vi "CIMAQ_distance_map.vi"(7 "size_x":u16=2000, 11 "size_y":u16=1000) -> (3 "distance_map":dbl[][](array[numeric]))   [LabVIEW 2014]
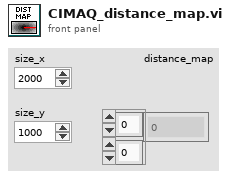
[diagram p1: front panel]
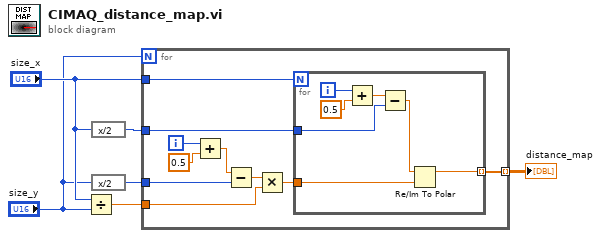
[diagram p0: block diagram]
diagram:
  n1 = Divide(x="size_x", y="size_y") -> (x/y=w5:dbl)
  n2 = expression code="x/2"("size_x") -> (w4:u16)
  n3 = expression code="x/2"("size_y") -> (w3:u16)
  n4 = for {
    N: "size_y" -> [_]
    tunnel: [w16] -> w6 mode=indexing
    tunnel: "size_x" -> [w15]
    tunnel: w5 -> [w12]
    tunnel: w4 -> [w11]
    tunnel: w3 -> [w10]
    i -> [w9]
    n5 = Add(x=w9, y=0.5 ("x*y")) -> (x+y=w7:dbl)
    n6 = Subtract(x=w7, y=w10) -> (x-y=w14:dbl)
    n7 = Multiply(x=w14, y=w12) -> (x*y=w13:dbl)
    n8 = for {
      N: w15 -> [_]
      tunnel: [w17] -> w16 mode=indexing
      tunnel: w13 -> [w22]
      tunnel: w11 -> [w21]
      i -> [w20]
      n9 = Add(x=w20, y=0.5 ("x*y")) -> (x+y=w19:dbl)
      n10 = Subtract(x=w19, y=w21) -> (x-y=w23:dbl)
      n11 = Re/Im To Polar(2:w22, 3:w23) -> (1:w17:dbl)  [unwired: 1 out]
    }
  }
  "distance_map" <- w6
